vi "NI9482_simpleUI.vi"() -> ()   [LabVIEW 2020]
uses:
  TYPEDEF/NI9482_TD_Method.ctl
panel:
  in  "Stop":bool
  in  "RLY":bool[](array[boolean])
  in  "Line(s)NI9482":tag="cDAQ1Mod1/port0/line0:3"
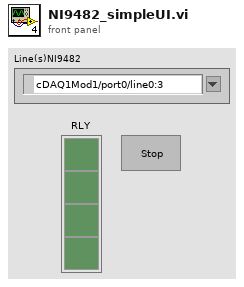
[diagram p1: front panel]
types:
  T1 = typedef "NI9482_TD_Method.ctl" = enum16{"NO_OP", "INIT", "SET", "CLOSE", "END"}
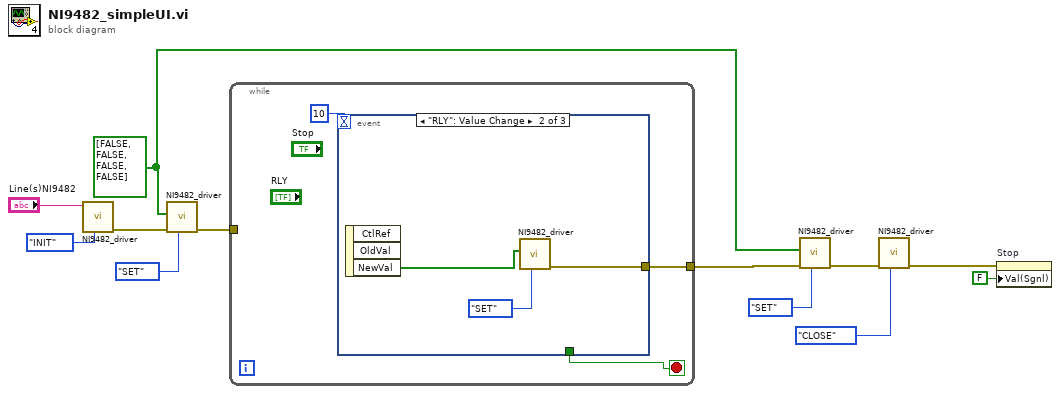
[diagram p0: block diagram]
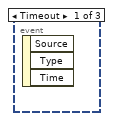
[diagram p2: hidden frame]
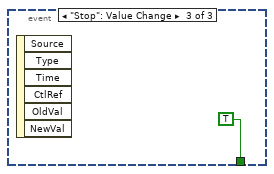
[diagram p3: hidden frame]
diagram:
  w5 = bool[] [FALSE, FALSE, FALSE, FALSE] ("Data 4 RLY")
  n1 = call "NI9482_driver.vi"("MethodNI9482"=NI9482_TD_Method."INIT", "Line(s)NI9482"="Line(s)NI9482") -> ("error out"=w10:errorcluster)  [unwired: 8 in, 1 out]
  n2 = call "NI9482_driver.vi"("MethodNI9482"=NI9482_TD_Method."SET", "error in (no error)"=w10, "Data 4 RLY"=w5) -> ("error out"=w8:errorcluster)  [unwired: 7 in, 1 out]
  n3 = while {
    tunnel: w8 -> [_]
    tunnel: [w13] -> w6
    stop <- w15 stop-if-true
    n4 = event shown="[1] \"RLY\": Value Change" {
      selector: _ -> [_ _ _]
      dyn-events: _ -> [_ _ _]
      timeout: 10 -> [_ _ _]
      tunnel: [_ w16 _] -> w13
      tunnel: [_ _ TRUE] -> w15
      event Timeout {
        n5 = event-data() -> ()  [unwired: 1 in, 3 out]
      }
      event "RLY": Value Change {
        n6 = event-data() -> ("NewVal"=w17:bool[])  [unwired: 1 in, 2 out]
        n7 = call "NI9482_driver.vi"("MethodNI9482"=NI9482_TD_Method."SET", "Data 4 RLY"=w17) -> ("error out"=w16:errorcluster)  [unwired: 8 in, 1 out]
      }
      event "Stop": Value Change {
        n8 = event-data() -> ()  [unwired: 1 in, 6 out]
      }
    }
  }
  n9 = call "NI9482_driver.vi"("MethodNI9482"=NI9482_TD_Method."SET", "error in (no error)"=w6, "Data 4 RLY"=w5) -> ("error out"=w2:errorcluster)  [unwired: 7 in, 1 out]
  n10 = call "NI9482_driver.vi"("MethodNI9482"=NI9482_TD_Method."CLOSE", "error in (no error)"=w2) -> ("error out"=w1:errorcluster)  [unwired: 8 in, 1 out]
  n11 = property on="Stop" class="Bool (strict)"(error in=w1, "Val(Sgnl)"=FALSE ("Value (Signaling)")) -> ()  [unwired: 1 in, 2 out]
